vi "Test - Draw Teapot.vi"() -> ()   [LabVIEW 2022 SP3, in "Raster.lvlib"] (continued)
 "Alpha Blending Enabled"=FALSE, "Colour"=131841}, {"Vertex 1"={"Position"={"x"=297.17767, "y"=396.39102, "z"=0.98972005}, "UV"={"u"=0.0, "v"=0.0}, "Colour"=12517256}, "Vertex 2"={"Position"={"x"=313.01276, "y"=398.35367, "z"=0.9897707}, "UV"={"u"=0.0, "v"=0.0}, "Colour"=12517256}, "Vertex 3"={"Position"={"x"=314.0461, "y"=401.00818, "z"=0.9894933}, "UV"={"u"=0.0, "v"=0.0}, "Colour"=12517256}, "Alpha"=0.0, "Alpha Blending Enabled"=FALSE, "Colour"=9091426}, {"Vertex 1"={"Position"={"x"=719.345, "y"=369.09378, "z"=0.9897083}, "UV"={"u"=0.0, "v"=0.0}, "Colour"=12517256}, "Vertex 2"={"Position"={"x"=706.15826, "y"=351.93036, "z"=0.9896661}, "UV"={"u"=0.0, "v"=0.0}, "Colour"=12517256}, "Vertex 3"={"Position"={"x"=702.0343, "y"=353.5881, "z"=0.98960906}, "UV"={"u"=0.0, "v"=0.0}, "Colour"=12517256}, "Alpha"=0.0, "Alpha Blending Enabled"=FALSE, "Colour"=5995329}, {"Vertex 1"={"Position"={"x"=682.03534, "y"=357.63016, "z"=0.9896661}, "UV"={"u"=0.0, "v"=0.0}, "Colour"=12517256}, "Vertex 2"={"Position"={"x"=677.0391, "y"=342.4919, "z"=0.9896034}, "UV"={"u"=0.0, "v"=0.0}, "Colour"=12517256}, "Vertex 3"={"Position"={"x"=669.9876, "y"=344.076, "z"=0.9897131}, "UV"={"u"=0.0, "v"=0.0}, "Colour"=12517256}, "Alpha"=0.0, "Alpha Blending Enabled"=FALSE, "Colour"=9354853}, {"Vertex 1"={"Position"={"x"=402.95343, "y"=420.3544, "z"=0.98970723}, "UV"={"u"=0.0, "v"=0.0}, "Colour"=12517256}, "Vertex 2"={"Position"={"x"=403.55054, "y"=415.85388, "z"=0.98963785}, "UV"={"u"=0.0, "v"=0.0}, "Colour"=12517256}, "Vertex 3"={"Position"={"x"=400.0, "y"=415.91602, "z"=0.9896323}, "UV"={"u"=0.0, "v"=0.0}, "Colour"=12517256}, "Alpha"=0.0, "Alpha Blending Enabled"=FALSE, "Colour"=12253573}, {"Vertex 1"={"Position"={"x"=221.27509, "y"=350.14075, "z"=0.9894772}, "UV"={"u"=0.0, "v"=0.0}, "Colour"=12517256}, "Vertex 2"={"Position"={"x"=213.20128, "y"=333.07422, "z"=0.9894514}, "UV"={"u"=0.0, "v"=0.0}, "Colour"=12517256}, "Vertex 3"={"Position"={"x"=221.4342, "y"=331.2093, "z"=0.990049}, "UV"={"u"=0.0, "v"=0.0}, "Colour"=12517256}, "Alpha"=0.0, "Alpha Blending Enabled"=FALSE, "Colour"=4282158}, {"Vertex 1"={"Position"={"x"=586.7987, "y"=333.07422, "z"=0.9894514}, "UV"={"u"=0.0, "v"=0.0}, "Colour"=12517256}, "Vertex 2"={"Position"={"x"=578.7249, "y"=350.14075, "z"=0.9894772}, "UV"={"u"=0.0, "v"=0.0}, "Colour"=12517256}, "Vertex 3"={"Position"={"x"=571.2652, "y"=347.42908, "z"=0.990049}, "UV"={"u"=0.0, "v"=0.0}, "Colour"=12517256}, "Alpha"=0.0, "Alpha Blending Enabled"=FALSE, "Colour"=4282158}, {"Vertex 1"={"Position"={"x"=373.0144, "y"=460.57834, "z"=0.9896675}, "UV"={"u"=0.0, "v"=0.0}, "Colour"=12517256}, "Vertex 2"={"Position"={"x"=368.50552, "y"=457.60767, "z"=0.98960376}, "UV"={"u"=0.0, "v"=0.0}, "Colour"=12517256}, "Vertex 3"={"Position"={"x"=365.71857, "y"=456.0784, "z"=0.9897051}, "UV"={"u"=0.0, "v"=0.0}, "Colour"=12517256}, "Alpha"=0.0, "Alpha Blending Enabled"=FALSE, "Colour"=9881963}, {"Vertex 1"={"Position"={"x"=706.8331, "y"=370.62793, "z"=0.9896408}, "UV"={"u"=0.0, "v"=0.0}, "Colour"=12517256}, "Vertex 2"={"Position"={"x"=723.916, "y"=383.22333, "z"=0.9896593}, "UV"={"u"=0.0, "v"=0.0}, "Colour"=12517256}, "Vertex 3"={"Position"={"x"=732.98505, "y"=383.09384, "z"=0.9896755}, "UV"={"u"=0.0, "v"=0.0}, "Colour"=12517256}, "Alpha"=0.0, "Alpha Blending Enabled"=FALSE, "Colour"=8432732}, {"Vertex 1"={"Position"={"x"=702.0343, "y"=353.5881, "z"=0.98960906}, "UV"={"u"=0.0, "v"=0.0}, "Colour"=12517256}, "Vertex 2"={"Position"={"x"=713.92786, "y"=369.94937, "z"=0.9896577}, "UV"={"u"=0.0, "v"=0.0}, "Colour"=12517256}, "Vertex 3"={"Position"={"x"=719.345, "y"=369.09378, "z"=0.9897083}, "UV"={"u"=0.0, "v"=0.0}, "Colour"=12517256}, "Alpha"=0.0, "Alpha Blending Enabled"=FALSE, "Colour"=7115086}, {"Vertex 1"={"Position"={"x"=391.0851, "y"=426.15314, "z"=0.9897195}, "UV"={"u"=0.0, "v"=0.0}, "Colour"=12517256}, "Vertex 2"={"Position"={"x"=388.97626, "y"=433.47845, "z"=0.9896417}, "UV"={"u"=0.0, "v"=0.0}, "Colour"=12517256}, "Vertex 3"={"Position"={"x"=392.3791, "y"=433.84442, "z"=0.9896132}, "UV"={"u"=0.0, "v"=0.0}, "Colour"=12517256}, "Alpha"=0.0, "Alpha Blending Enabled"=FALSE, "Colour"=1712915}, {"Vertex 1"={"Position"={"x"=396.07202, "y"=434.0735, "z"=0.9895953}, "UV"={"u"=0.0, "v"=0.0}, "Colour"=12517256}, "Vertex 2"={"Position"={"x"=396.8272, "y"=426.60828, "z"=0.9896822}, "UV"={"u"=0.0, "v"=0.0}, "Colour"=12517256}, "Vertex 3"={"Position"={"x"=393.84116, "y"=426.43307, "z"=0.98969656}, "UV"={"u"=0.0, "v"=0.0}, "Colour"=12517256}, "Alpha"=0.0, "Alpha Blending Enabled"=FALSE, "Colour"=2107927}, {"Vertex 1"={"Position"={"x"=732.98505, "y"=383.09384, "z"=0.9896755}, "UV"={"u"=0.0, "v"=0.0}, "Colour"=12517256}, "Vertex 2"={"Position"={"x"=713.92786, "y"=369.94937, "z"=0.9896577}, "UV"={"u"=0.0, "v"=0.0}, "Colour"=12517256}, "Vertex 3"={"Position"={"x"=706.8331, "y"=370.62793, "z"=0.9896408}, "UV"={"u"=0.0, "v"=0.0}, "Colour"=12517256}, "Alpha"=0.0, "Alpha Blending Enabled"=FALSE, "Colour"=7971671}, {"Vertex 1"={"Position"={"x"=400.0, "y"=420.40808, "z"=0.9897026}, "UV"={"u"=0.0, "v"=0.0}, "Colour"=12517256}, "Vertex 2"={"Position"={"x"=400.0, "y"=415.91602, "z"=0.9896323}, "UV"={"u"=0.0, "v"=0.0}, "Colour"=12517256}, "Vertex 3"={"Position"={"x"=396.44946, "y"=415.85388, "z"=0.98963785}, "UV"={"u"=0.0, "v"=0.0}, "Colour"=12517256}, "Alpha"=0.0, "Alpha Blending Enabled"=FALSE, "Colour"=12253573}, {"Vertex 1"={"Position"={"x"=666.5026, "y"=329.28787, "z"=0.9896555}, "UV"={"u"=0.0, "v"=0.0}, "Colour"=12517256}, "Vertex 2"={"Position"={"x"=669.9876, "y"=344.076, "z"=0.9897131}, "UV"={"u"=0.0, "v"=0.0}, "Colour"=12517256}, "Vertex 3"={"Position"={"x"=677.0391, "y"=342.4919, "z"=0.9896034}, "UV"={"u"=0.0, "v"=0.0}, "Colour"=12517256}, "Alpha"=0.0, "Alpha Blending Enabled"=FALSE, "Colour"=8827744}, {"Vertex 1"={"Position"={"x"=381.9381, "y"=412.10922, "z"=0.98957527}, "UV"={"u"=0.0, "v"=0.0}, "Colour"=12517256}, "Vertex 2"={"Position"={"x"=387.2426, "y"=415.00214, "z"=0.98971444}, "UV"={"u"=0.0, "v"=0.0}, "Colour"=12517256}, "Vertex 3"={"Position"={"x"=390.02243, "y"=415.3864, "z"=0.9896799}, "UV"={"u"=0.0, "v"=0.0}, "Colour"=12517256}, "Alpha"=0.0, "Alpha Blending Enabled"=FALSE, "Colour"=11331451}, {"Vertex 1"={"Position"={"x"=415.18842, "y"=414.5321, "z"=0.9897567}, "UV"={"u"=0.0, "v"=0.0}, "Colour"=12517256}, "Vertex 2"={"Position"={"x"=421.46735, "y"=411.46152, "z"=0.9896358}, "UV"={"u"=0.0, "v"=0.0}, "Colour"=12517256}, "Vertex 3"={"Position"={"x"=418.06192, "y"=412.10922, "z"=0.98957527}, "UV"={"u"=0.0, "v"=0.0}, "Colour"=12517256}, "Alpha"=0.0, "Alpha Blending Enabled"=FALSE, "Colour"=10936183}, {"Vertex 1"={"Position"={"x"=678.03265, "y"=257.92834, "z"=0.98976254}, "UV"={"u"=0.0, "v"=0.0}, "Colour"=12517256}, "Vertex 2"={"Position"={"x"=666.5512, "y"=236.05386, "z"=0.9897306}, "UV"={"u"=0.0, "v"=0.0}, "Colour"=12517256}, "Vertex 3"={"Position"={"x"=671.18396, "y"=239.12437, "z"=0.9894685}, "UV"={"u"=0.0, "v"=0.0}, "Colour"=12517256}, "Alpha"=0.0, "Alpha Blending Enabled"=FALSE, "Colour"=131841}, {"Vertex 1"={"Position"={"x"=723.916, "y"=383.22333, "z"=0.9896593}, "UV"={"u"=0.0, "v"=0.0}, "Colour"=12517256}, "Vertex 2"={"Position"={"x"=706.8331, "y"=370.62793, "z"=0.9896408}, "UV"={"u"=0.0, "v"=0.0}, "Colour"=12517256}, "Vertex 3"={"Position"={"x"=698.73804, "y"=371.07614, "z"=0.9896577}, "UV"={"u"=0.0, "v"=0.0}, "Colour"=12517256}, "Alpha"=0.0, "Alpha Blending Enabled"=FALSE, "Colour"=10409073}, {"Vertex 1"={"Position"={"x"=383.24374, "y"=432.39114, "z"=0.98972654}, "UV"={"u"=0.0, "v"=0.0}, "Colour"=12517256}, "Vertex 2"={"Position"={"x"=378.97202, "y"=439.917, "z"=0.9896443}, "UV"={"u"=0.0, "v"=0.0}, "Colour"=12517256}, "Vertex 3"={"Position"={"x"=382.30276, "y"=440.7109, "z"=0.9895852}, "UV"={"u"=0.0, "v"=0.0}, "Colour"=12517256}, "Alpha"=0.0, "Alpha Blending Enabled"=FALSE, "Colour"=131841}, {"Vertex 1"={"Position"={"x"=209.53932, "y"=162.75063, "z"=0.9894397}, "UV"={"u"=0.0, "v"=0.0}, "Colour"=12517256}, "Vertex 2"={"Position"={"x"=218.06183, "y"=155.67198, "z"=0.9894669}, "UV"={"u"=0.0, "v"=0.0}, "Colour"=12517256}, "Vertex 3"={"Position"={"x"=225.82498, "y"=163.60995, "z"=0.990049}, "UV"={"u"=0.0, "v"=0.0}, "Colour"=12517256}, "Alpha"=0.0, "Alpha Blending Enabled"=FALSE, "Colour"=131841}, {"Vertex 1"={"Position"={"x"=581.9382, "y"=155.67198, "z"=0.9894669}, "UV"={"u"=0.0, "v"=0.0}, "Colour"=12517256}, "Vertex 2"={"Position"={"x"=590.4607, "y"=162.75063, "z"=0.9894397}, "UV"={"u"=0.0, "v"=0.0}, "Colour"=12517256}, "Vertex 3"={"Position"={"x"=581.86536, "y"=170.63258, "z"=0.990049}, "UV"={"u"=0.0, "v"=0.0}, "Colour"=12517256}, "Alpha"=0.0, "Alpha Blending Enabled"=FALSE, "Colour"=131841}, {"Vertex 1"={"Position"={"x"=428.45627, "y"=446.1597, "z"=0.9896467}, "UV"={"u"=0.0, "v"=0.0}, "Colour"=12517256}, "Vertex 2"={"Position"={"x"=431.51227, "y"=452.57986, "z"=0.9896035}, "UV"={"u"=0.0, "v"=0.0}, "Colour"=12517256}, "Vertex 3"={"Position"={"x"=434.30084, "y"=451.0985, "z"=0.98970497}, "UV"={"u"=0.0, "v"=0.0}, "Colour"=12517256}, "Alpha"=0.0, "Alpha Blending Enabled"=FALSE, "Colour"=131841}, {"Vertex 1"={"Position"={"x"=403.92798, "y"=434.0735, "z"=0.9895953}, "UV"={"u"=0.0, "v"=0.0}, "Colour"=12517256}, "Vertex 2"={"Position"={"x"=403.1728, "y"=426.60828, "z"=0.9896822}, "UV"={"u"=0.0, "v"=0.0}, "Colour"=12517256}, "Vertex 3"={"Position"={"x"=400.0, "y"=426.66876, "z"=0.98967725}, "UV"={"u"=0.0, "v"=0.0}, "Colour"=12517256}, "Alpha"=0.0, "Alpha Blending Enabled"=FALSE, "Colour"=2240025}, {"Vertex 1"={"Position"={"x"=406.1588, "y"=426.43307, "z"=0.98969656}, "UV"={"u"=0.0, "v"=0.0}, "Colour"=12517256}, "Vertex 2"={"Position"={"x"=407.6209, "y"=433.84442, "z"=0.9896132}, "UV"={"u"=0.0, "v"=0.0}, "Colour"=12517256}, "Vertex 3"={"Position"={"x"=411.0237, "y"=433.47845, "z"=0.9896417}, "UV"={"u"=0.0, "v"=0.0}, "Colour"=12517256}, "Alpha"=0.0, "Alpha Blending Enabled"=FALSE, "Colour"=1712915}, {"Vertex 1"={"Position"={"x"=400.0, "y"=434.1526, "z"=0.9895892}, "UV"={"u"=0.0, "v"=0.0}, "Colour"=12517256}, "Vertex 2"={"Position"={"x"=400.0, "y"=426.66876, "z"=0.98967725}, "UV"={"u"=0.0, "v"=0.0}, "Colour"=12517256}, "Vertex 3"={"Position"={"x"=396.8272, "y"=426.60828, "z"=0.9896822}, "UV"={"u"=0.0, "v"=0.0}, "Colour"=12517256}, "Alpha"=0.0, "Alpha Blending Enabled"=FALSE, "Colour"=2240025}, {"Vertex 1"={"Position"={"x"=326.15854, "y"=127.58133, "z"=0.9898128}, "UV"={"u"=0.0, "v"=0.0}, "Colour"=12517256}, "Vertex 2"={"Position"={"x"=299.14365, "y"=127.179695, "z"=0.98972636}, "UV"={"u"=0.0, "v"=0.0}, "Colour"=12517256}, "Vertex 3"={"Position"={"x"=299.91116, "y"=121.74838, "z"=0.98940194}, "UV"={"u"=0.0, "v"=0.0}, "Colour"=12517256}, "Alpha"=0.0, "Alpha Blending Enabled"=FALSE, "Colour"=131841}, {"Vertex 1"={"Position"={"x"=375.695, "y"=410.7137, "z"=0.9897057}, "UV"={"u"=0.0, "v"=0.0}, "Colour"=12517256}, "Vertex 2"={"Position"={"x"=365.49564, "y"=408.5937, "z"=0.9895617}, "UV"={"u"=0.0, "v"=0.0}, "Colour"=12517256}, "Vertex 3"={"Position"={"x"=362.46423, "y"=407.4392, "z"=0.98967314}, "UV"={"u"=0.0, "v"=0.0}, "Colour"=12517256}, "Alpha"=0.0, "Alpha Blending Enabled"=FALSE, "Colour"=9816171}, {"Vertex 1"={"Position"={"x"=379.9003, "y"=462.82288, "z"=0.98952234}, "UV"={"u"=0.0, "v"=0.0}, "Colour"=12517256}, "Vertex 2"={"Position"={"x"=387.57538, "y"=462.27194, "z"=0.98972344}, "UV"={"u"=0.0, "v"=0.0}, "Colour"=12517256}, "Vertex 3"={"Position"={"x"=390.27826, "y"=462.79736, "z"=0.98969}, "UV"={"u"=0.0, "v"=0.0}, "Colour"=12517256}, "Alpha"=0.0, "Alpha Blending Enabled"=FALSE, "Colour"=10211439}, {"Vertex 1"={"Position"={"x"=698.73804, "y"=371.07614, "z"=0.9896577}, "UV"={"u"=0.0, "v"=0.0}, "Colour"=12517256}, "Vertex 2"={"Position"={"x"=689.394, "y"=356.5748, "z"=0.98960906}, "UV"={"u"=0.0, "v"=0.0}, "Colour"=12517256}, "Vertex 3"={"Position"={"x"=682.03534, "y"=357.63016, "z"=0.9896661}, "UV"={"u"=0.0, "v"=0.0}, "Colour"=12517256}, "Alpha"=0.0, "Alpha Blending Enabled"=FALSE, "Colour"=11001976}, {"Vertex 1"={"Position"={"x"=213.20128, "y"=333.07422, "z"=0.9894514}, "UV"={"u"=0.0, "v"=0.0}, "Colour"=12517256}, "Vertex 2"={"Position"={"x"=205.60883, "y"=316.07062, "z"=0.9894271}, "UV"={"u"=0.0, "v"=0.0}, "Colour"=12517256}, "Vertex 3"={"Position"={"x"=214.60127, "y"=315.1298, "z"=0.990049}, "UV"={"u"=0.0, "v"=0.0}, "Colour"=12517256}, "Alpha"=0.0, "Alpha Blending Enabled"=FALSE, "Colour"=4084524}, {"Vertex 1"={"Position"={"x"=594.3912, "y"=316.07062, "z"=0.9894271}, "UV"={"u"=0.0, "v"=0.0}, "Colour"=12517256}, "Vertex 2"={"Position"={"x"=586.7987, "y"=333.07422, "z"=0.9894514}, "UV"={"u"=0.0, "v"=0.0}, "Colour"=12517256}, "Vertex 3"={"Position"={"x"=578.5658, "y"=331.2093, "z"=0.990049}, "UV"={"u"=0.0, "v"=0.0}, "Colour"=12517256}, "Alpha"=0.0, "Alpha Blending Enabled"=FALSE, "Colour"=4084524}, {"Vertex 1"={"Position"={"x"=387.2426, "y"=415.00214, "z"=0.98971444}, "UV"={"u"=0.0, "v"=0.0}, "Colour"=12517256}, "Vertex 2"={"Position"={"x"=381.9381, "y"=412.10922, "z"=0.98957527}, "UV"={"u"=0.0, "v"=0.0}, "Colour"=12517256}, "Vertex 3"={"Position"={"x"=378.53265, "y"=411.46152, "z"=0.9896358}, "UV"={"u"=0.0, "v"=0.0}, "Colour"=12517256}, "Alpha"=0.0, "Alpha Blending Enabled"=FALSE, "Colour"=10936183}, {"Vertex 1"={"Position"={"x"=376.19745, "y"=438.9993, "z"=0.9897126}, "UV"={"u"=0.0, "v"=0.0}, "Colour"=12517256}, "Vertex 2"={"Position"={"x"=371.54373, "y"=446.1597, "z"=0.9896467}, "UV"={"u"=0.0, "v"=0.0}, "Colour"=12517256}, "Vertex 3"={"Position"={"x"=374.82742, "y"=447.3146, "z"=0.98956454}, "UV"={"u"=0.0, "v"=0.0}, "Colour"=12517256}, "Alpha"=0.0, "Alpha Blending Enabled"=FALSE, "Colour"=131841}, {"Vertex 1"={"Position"={"x"=374.82742, "y"=447.3146, "z"=0.98956454}, "UV"={"u"=0.0, "v"=0.0}, "Colour"=12517256}, "Vertex 2"={"Position"={"x"=378.97202, "y"=439.917, "z"=0.9896443}, "UV"={"u"=0.0, "v"=0.0}, "Colour"=12517256}, "Vertex 3"={"Position"={"x"=376.19745, "y"=438.9993, "z"=0.9897126}, "UV"={"u"=0.0, "v"=0.0}, "Colour"=12517256}, "Alpha"=0.0, "Alpha Blending Enabled"=FALSE, "Colour"=131841}, {"Vertex 1"={"Position"={"x"=414.14594, "y"=412.64026, "z"=0.98952574}, "UV"={"u"=0.0, "v"=0.0}, "Colour"=12517256}, "Vertex 2"={"Position"={"x"=409.97757, "y"=415.3864, "z"=0.9896799}, "UV"={"u"=0.0, "v"=0.0}, "Colour"=12517256}, "Vertex 3"={"Position"={"x"=412.75735, "y"=415.00214, "z"=0.98971444}, "UV"={"u"=0.0, "v"=0.0}, "Colour"=12517256}, "Alpha"=0.0, "Alpha Blending Enabled"=FALSE, "Colour"=11331451}, {"Vertex 1"={"Position"={"x"=682.01483, "y"=260.7837, "z"=0.9895282}, "UV"={"u"=0.0, "v"=0.0}, "Colour"=12517256}, "Vertex 2"={"Position"={"x"=688.6595, "y"=283.87192, "z"=0.9895922}, "UV"={"u"=0.0, "v"=0.0}, "Colour"=12517256}, "Vertex 3"={"Position"={"x"=685.4334, "y"=281.3033, "z"=0.9897971}, "UV"={"u"=0.0, "v"=0.0}, "Colour"=12517256}, "Alpha"=0.0, "Alpha Blending Enabled"=FALSE, "Colour"=131841}, {"Vertex 1"={"Position"={"x"=485.95386, "y"=401.00818, "z"=0.9894933}, "UV"={"u"=0.0, "v"=0.0}, "Colour"=12517256}, "Vertex 2"={"Position"={"x"=469.47156, "y"=402.4644, "z"=0.9895999}, "UV"={"u"=0.0, "v"=0.0}, "Colour"=12517256}, "Vertex 3"={"Position"={"x"=470.66293, "y"=400.277, "z"=0.989823}, "UV"={"u"=0.0, "v"=0.0}, "Colour"=12517256}, "Alpha"=0.0, "Alpha Blending Enabled"=FALSE, "Colour"=9091426}, {"Vertex 1"={"Position"={"x"=431.51227, "y"=452.57986, "z"=0.9896035}, "UV"={"u"=0.0, "v"=0.0}, "Colour"=12517256}, "Vertex 2"={"Position"={"x"=431.49448, "y"=457.60767, "z"=0.98960376}, "UV"={"u"=0.0, "v"=0.0}, "Colour"=12517256}, "Vertex 3"={"Position"={"x"=434.28143, "y"=456.0784, "z"=0.9897051}, "UV"={"u"=0.0, "v"=0.0}, "Colour"=12517256}, "Alpha"=0.0, "Alpha Blending Enabled"=FALSE, "Colour"=4677427}, {"Vertex 1"={"Position"={"x"=362.46423, "y"=407.4392, "z"=0.98967314}, "UV"={"u"=0.0, "v"=0.0}, "Colour"=12517256}, "Vertex 2"={"Position"={"x"=348.88834, "y"=405.76608, "z"=0.98953724}, "UV"={"u"=0.0, "v"=0.0}, "Colour"=12517256}, "Vertex 3"={"Position"={"x"=346.3009, "y"=404.1098, "z"=0.98970187}, "UV"={"u"=0.0, "v"=0.0}, "Colour"=12517256}, "Alpha"=0.0, "Alpha Blending Enabled"=FALSE, "Colour"=9355110}, {"Vertex 1"={"Position"={"x"=368.50552, "y"=457.60767, "z"=0.98960376}, "UV"={"u"=0.0, "v"=0.0}, "Colour"=12517256}, "Vertex 2"={"Position"={"x"=368.48776, "y"=452.57986, "z"=0.9896035}, "UV"={"u"=0.0, "v"=0.0}, "Colour"=12517256}, "Vertex 3"={"Position"={"x"=365.69916, "y"=451.0985, "z"=0.98970497}, "UV"={"u"=0.0, "v"=0.0}, "Colour"=12517256}, "Alpha"=0.0, "Alpha Blending Enabled"=FALSE, "Colour"=4677427}, {"Vertex 1"={"Position"={"x"=192.4563, "y"=195.83786, "z"=0.9896561}, "UV"={"u"=0.0, "v"=0.0}, "Colour"=12517256}, "Vertex 2"={"Position"={"x"=171.12422, "y"=206.32034, "z"=0.9896561}, "UV"={"u"=0.0, "v"=0.0}, "Colour"=12517256}, "Vertex 3"={"Position"={"x"=169.41815, "y"=209.785, "z"=0.98959744}, "UV"={"u"=0.0, "v"=0.0}, "Colour"=12517256}, "Alpha"=0.0, "Alpha Blending Enabled"=FALSE, "Colour"=1515280}, {"Vertex 1"={"Position"={"x"=169.40346, "y"=222.90483, "z"=0.9896561}, "UV"={"u"=0.0, "v"=0.0}, "Colour"=12517256}, "Vertex 2"={"Position"={"x"=186.3216, "y"=214.24203, "z"=0.9896561}, "UV"={"u"=0.0, "v"=0.0}, "Colour"=12517256}, "Vertex 3"={"Position"={"x"=186.59279, "y"=209.32652, "z"=0.98959744}, "UV"={"u"=0.0, "v"=0.0}, "Colour"=12517256}, "Alpha"=0.0, "Alpha Blending Enabled"=FALSE, "Colour"=11858305}, {"Vertex 1"={"Position"={"x"=171.12422, "y"=206.32034, "z"=0.9896561}, "UV"={"u"=0.0, "v"=0.0}, "Colour"=12517256}, "Vertex 2"={"Position"={"x"=152.20497, "y"=217.41687, "z"=0.9896561}, "UV"={"u"=0.0, "v"=0.0}, "Colour"=12517256}, "Vertex 3"={"Position"={"x"=151.36185, "y"=220.60233, "z"=0.98959744}, "UV"={"u"=0.0, "v"=0.0}, "Colour"=12517256}, "Alpha"=0.0, "Alpha Blending Enabled"=FALSE, "Colour"=1778707}, {"Vertex 1"={"Position"={"x"=154.51155, "y"=232.58194, "z"=0.9896561}, "UV"={"u"=0.0, "v"=0.0}, "Colour"=12517256}, "Vertex 2"={"Position"={"x"=169.40346, "y"=222.90483, "z"=0.9896561}, "UV"={"u"=0.0, "v"=0.0}, "Colour"=12517256}, "Vertex 3"={"Position"={"x"=168.51642, "y"=218.47636, "z"=0.98959744}, "UV"={"u"=0.0, "v"=0.0}, "Colour"=12517256}, "Alpha"=0.0, "Alpha Blending Enabled"=FALSE, "Colour"=11529085}, {"Vertex 1"={"Position"={"x"=152.20497, "y"=217.41687, "z"=0.9896561}, "UV"={"u"=0.0, "v"=0.0}, "Colour"=12517256}, "Vertex 2"={"Position"={"x"=135.65894, "y"=229.04527, "z"=0.9896561}, "UV"={"u"=0.0, "v"=0.0}, "Colour"=12517256}, "Vertex 3"={"Position"={"x"=135.59482, "y"=232.01439, "z"=0.98959744}, "UV"={"u"=0.0, "v"=0.0}, "Colour"=12517256}, "Alpha"=0.0, "Alpha Blending Enabled"=FALSE, "Colour"=2240024}, {"Vertex 1"={"Position"={"x"=141.58824, "y"=243.03935, "z"=0.9896561}, "UV"={"u"=0.0, "v"=0.0}, "Colour"=12517256}, "Vertex 2"={"Position"={"x"=154.51155, "y"=232.58194, "z"=0.9896561}, "UV"={"u"=0.0, "v"=0.0}, "Colour"=12517256}, "Vertex 3"={"Position"={"x"=152.57072, "y"=228.54994, "z"=0.98959744}, "UV"={"u"=0.0, "v"=0.0}, "Colour"=12517256}, "Alpha"=0.0, "Alpha Blending Enabled"=FALSE, "Colour"=11199609}, {"Vertex 1"={"Position"={"x"=135.65894, "y"=229.04527, "z"=0.9896561}, "UV"={"u"=0.0, "v"=0.0}, "Colour"=12517256}, "Vertex 2"={"Position"={"x"=121.447014, "y"=241.12357, "z"=0.9896561}, "UV"={"u"=0.0, "v"=0.0}, "Colour"=12517256}, "Vertex 3"={"Position"={"x"=122.07298, "y"=243.90215, "z"=0.98959744}, "UV"={"u"=0.0, "v"=0.0}, "Colour"=12517256}, "Alpha"=0.0, "Alpha Blending Enabled"=FALSE, "Colour"=2898719}, {"Vertex 1"={"Position"={"x"=130.57544, "y"=254.04317, "z"=0.9896561}, "UV"={"u"=0.0, "v"=0.0}, "Colour"=12517256}, "Vertex 2"={"Position"={"x"=141.58824, "y"=243.03935, "z"=0.9896561}, "UV"={"u"=0.0, "v"=0.0}, "Colour"=12517256}, "Vertex 3"={"Position"={"x"=138.70209, "y"=239.3482, "z"=0.98959744}, "UV"={"u"=0.0, "v"=0.0}, "Colour"=12517256}, "Alpha"=0.0, "Alpha Blending Enabled"=FALSE, "Colour"=10804341}, {"Vertex 1"={"Position"={"x"=121.447014, "y"=241.12357, "z"=0.9896561}, "UV"={"u"=0.0, "v"=0.0}, "Colour"=12517256}, "Vertex 2"={"Position"={"x"=109.52954, "y"=253.56958, "z"=0.9896561}, "UV"={"u"=0.0, "v"=0.0}, "Colour"=12517256}, "Vertex 3"={"Position"={"x"=110.75225, "y"=256.14658, "z"=0.98959744}, "UV"={"u"=0.0, "v"=0.0}, "Colour"=12517256}, "Alpha"=0.0, "Alpha Blending Enabled"=FALSE, "Colour"=3557415}, {"Vertex 1"={"Position"={"x"=121.415565, "y"=265.35983, "z"=0.9896561}, "UV"={"u"=0.0, "v"=0.0}, "Colour"=12517256}, "Vertex 2"={"Position"={"x"=130.57544, "y"=254.04317, "z"=0.9896561}, "UV"={"u"=0.0, "v"=0.0}, "Colour"=12517256}, "Vertex 3"={"Position"={"x"=126.85683, "y"=250.67299, "z"=0.98959744}, "UV"={"u"=0.0, "v"=0.0}, "Colour"=12517256}, "Alpha"=0.0, "Alpha Blending Enabled"=FALSE, "Colour"=10409073}, {"Vertex 1"={"Position"={"x"=109.52954, "y"=253.56958, "z"=0.9896561}, "UV"={"u"=0.0, "v"=0.0}, "Colour"=12517256}, "Vertex 2"={"Position"={"x"=99.86725, "y"=266.30142, "z"=0.9896561}, "UV"={"u"=0.0, "v"=0.0}, "Colour"=12517256}, "Vertex 3"={"Position"={"x"=101.588585, "y"=268.6284, "z"=0.98959744}, "UV"={"u"=0.0, "v"=0.0}, "Colour"=12517256}, "Alpha"=0.0, "Alpha Blending Enabled"=FALSE, "Colour"=4216366}, {"Vertex 1"={"Position"={"x"=114.0508, "y"=276.7551, "z"=0.9896561}, "UV"={"u"=0.0, "v"=0.0}, "Colour"=12517256}, "Vertex 2"={"Position"={"x"=121.415565, "y"=265.35983, "z"=0.9896561}, "UV"={"u"=0.0, "v"=0.0}, "Colour"=12517256}, "Vertex 3"={"Position"={"x"=116.981316, "y"=262.32532, "z"=0.98959744}, "UV"={"u"=0.0, "v"=0.0}, "Colour"=12517256}, "Alpha"=0.0, "Alpha Blending Enabled"=FALSE, "Colour"=9948012}, {"Vertex 1"={"Position"={"x"=99.86725, "y"=266.30142, "z"=0.9896561}, "UV"={"u"=0.0, "v"=0.0}, "Colour"=12517256}, "Vertex 2"={"Position"={"x"=92.42079, "y"=279.23703, "z"=0.9896561}, "UV"={"u"=0.0, "v"=0.0}, "Colour"=12517256}, "Vertex 3"={"Position"={"x"=94.53805, "y"=281.22873, "z"=0.98959744}, "UV"={"u"=0.0, "v"=0.0}, "Colour"=12517256}, "Alpha"=0.0, "Alpha Blending Enabled"=FALSE, "Colour"=4940853}, {"Vertex 1"={"Position"={"x"=108.42314, "y"=287.9951, "z"=0.9896561}, "UV"={"u"=0.0, "v"=0.0}, "Colour"=12517256}, "Vertex 2"={"Position"={"x"=114.0508, "y"=276.7551, "z"=0.9896561}, "UV"={"u"=0.0, "v"=0.0}, "Colour"=12517256}, "Vertex 3"={"Position"={"x"=109.02176, "y"=274.10672, "z"=0.98959744}, "UV"={"u"=0.0, "v"=0.0}, "Colour"=12517256}, "Alpha"=0.0, "Alpha Blending Enabled"=FALSE, "Colour"=9552487}, {"Vertex 1"={"Position"={"x"=92.42079, "y"=279.23703, "z"=0.9896561}, "UV"={"u"=0.0, "v"=0.0}, "Colour"=12517256}, "Vertex 2"={"Position"={"x"=87.15057, "y"=292.2944, "z"=0.9896561}, "UV"={"u"=0.0, "v"=0.0}, "Colour"=12517256}, "Vertex 3"={"Position"={"x"=89.5565, "y"=293.82855, "z"=0.98959744}, "UV"={"u"=0.0, "v"=0.0}, "Colour"=12517256}, "Alpha"=0.0, "Alpha Blending Enabled"=FALSE, "Colour"=5599805}, {"Vertex 1"={"Position"={"x"=104.47511, "y"=298.84622, "z"=0.9896561}, "UV"={"u"=0.0, "v"=0.0}, "Colour"=12517256}, "Vertex 2"={"Position"={"x"=108.42314, "y"=287.9951, "z"=0.9896561}, "UV"={"u"=0.0, "v"=0.0}, "Colour"=12517256}, "Vertex 3"={"Position"={"x"=102.92444, "y"=285.8186, "z"=0.98959744}, "UV"={"u"=0.0, "v"=0.0}, "Colour"=12517256}, "Alpha"=0.0, "Alpha Blending Enabled"=FALSE, "Colour"=9025634}, {"Vertex 1"={"Position"={"x"=87.15057, "y"=292.2944, "z"=0.9896561}, "UV"={"u"=0.0, "v"=0.0}, "Colour"=12517256}, "Vertex 2"={"Position"={"x"=84.01742, "y"=305.39136, "z"=0.9896561}, "UV"={"u"=0.0, "v"=0.0}, "Colour"=12517256}, "Vertex 3"={"Position"={"x"=86.5999, "y"=306.30865, "z"=0.98959744}, "UV"={"u"=0.0, "v"=0.0}, "Colour"=12517256}, "Alpha"=0.0, "Alpha Blending Enabled"=FALSE, "Colour"=6258756}, {"Vertex 1"={"Position"={"x"=102.14853, "y"=309.0745, "z"=0.9896561}, "UV"={"u"=0.0, "v"=0.0}, "Colour"=12517256}, "Vertex 2"={"Position"={"x"=104.47511, "y"=298.84622, "z"=0.9896561}, "UV"={"u"=0.0, "v"=0.0}, "Colour"=12517256}, "Vertex 3"={"Position"={"x"=98.63565, "y"=297.2621, "z"=0.98959744}, "UV"={"u"=0.0, "v"=0.0}, "Colour"=12517256}, "Alpha"=0.0, "Alpha Blending Enabled"=FALSE, "Colour"=8432732}, {"Vertex 1"={"Position"={"x"=84.01742, "y"=305.39136, "z"=0.9896561}, "UV"={"u"=0.0, "v"=0.0}, "Colour"=12517256}, "Vertex 2"={"Position"={"x"=82.98175, "y"=318.44592, "z"=0.9896561}, "UV"={"u"=0.0, "v"=0.0}, "Colour"=12517256}, "Vertex 3"={"Position"={"x"=85.62412, "y"=318.55002, "z"=0.98959744}, "UV"={"u"=0.0, "v"=0.0}, "Colour"=12517256}, "Alpha"=0.0, "Alpha Blending Enabled"=FALSE, "Colour"=6983244}, {"Vertex 1"={"Position"={"x"=101.3859, "y"=318.44592, "z"=0.9896561}, "UV"={"u"=0.0, "v"=0.0}, "Colour"=12517256}, "Vertex 2"={"Position"={"x"=102.14853, "y"=309.0745, "z"=0.9896561}, "UV"={"u"=0.0, "v"=0.0}, "Colour"=12517256}, "Vertex 3"={"Position"={"x"=96.10178, "y"=308.23883, "z"=0.98959744}, "UV"={"u"=0.0, "v"=0.0}, "Colour"=12517256}, "Alpha"=0.0, "Alpha Blending Enabled"=FALSE, "Colour"=7773780}, {"Vertex 1"={"Position"={"x"=82.98175, "y"=318.44592, "z"=0.9896561}, "UV"={"u"=0.0, "v"=0.0}, "Colour"=12517256}, "Vertex 2"={"Position"={"x"=84.52947, "y"=330.19464, "z"=0.9896561}, "UV"={"u"=0.0, "v"=0.0}, "Colour"=12517256}, "Vertex 3"={"Position"={"x"=87.13484, "y"=329.46445, "z"=0.98959744}, "UV"={"u"=0.0, "v"=0.0}, "Colour"=12517256}, "Alpha"=0.0, "Alpha Blending Enabled"=FALSE, "Colour"=8037463}, {"Vertex 1"={"Position"={"x"=102.74355, "y"=326.45404, "z"=0.9896561}, "UV"={"u"=0.0, "v"=0.0}, "Colour"=12517256}, "Vertex 2"={"Position"={"x"=101.3859, "y"=318.44592, "z"=0.9896561}, "UV"={"u"=0.0, "v"=0.0}, "Colour"=12517256}, "Vertex 3"={"Position"={"x"=95.26916, "y"=318.55002, "z"=0.98959744}, "UV"={"u"=0.0, "v"=0.0}, "Colour"=12517256}, "Alpha"=0.0, "Alpha Blending Enabled"=FALSE, "Colour"=6522183}, {"Vertex 1"={"Position"={"x"=84.52947, "y"=330.19464, "z"=0.9896561}, "UV"={"u"=0.0, "v"=0.0}, "Colour"=12517256}, "Vertex 2"={"Position"={"x"=89.163445, "y"=339.60242, "z"=0.9896561}, "UV"={"u"=0.0, "v"=0.0}, "Colour"=12517256}, "Vertex 3"={"Position"={"x"=91.65158, "y"=338.20395, "z"=0.98959744}, "UV"={"u"=0.0, "v"=0.0}, "Colour"=12517256}, "Alpha"=0.0, "Alpha Blending Enabled"=FALSE, "Colour"=9552744}, {"Vertex 1"={"Position"={"x"=106.78244, "y"=332.86646, "z"=0.9896561}, "UV"={"u"=0.0, "v"=0.0}, "Colour"=12517256}, "Vertex 2"={"Position"={"x"=102.74355, "y"=326.45404, "z"=0.9896561}, "UV"={"u"=0.0, "v"=0.0}, "Colour"=12517256}, "Vertex 3"={"Position"={"x"=96.68016, "y"=327.50403, "z"=0.98959744}, "UV"={"u"=0.0, "v"=0.0}, "Colour"=12517256}, "Alpha"=0.0, "Alpha Blending Enabled"=FALSE, "Colour"=4545841}, {"Vertex 1"={"Position"={"x"=89.163445, "y"=339.60242, "z"=0.9896561}, "UV"={"u"=0.0, "v"=0.0}, "Colour"=12517256}, "Vertex 2"={"Position"={"x"=96.86964, "y"=346.92914, "z"=0.9896561}, "UV"={"u"=0.0, "v"=0.0}, "Colour"=12517256}, "Vertex 3"={"Position"={"x"=99.15168, "y"=345.0104, "z"=0.98959744}, "UV"={"u"=0.0, "v"=0.0}, "Colour"=12517256}, "Alpha"=0.0, "Alpha Blending Enabled"=FALSE, "Colour"=10936183}, {"Vertex 1"={"Position"={"x"=113.45179, "y"=337.86047, "z"=0.9896561}, "UV"={"u"=0.0, "v"=0.0}, "Colour"=12517256}, "Vertex 2"={"Position"={"x"=106.78244, "y"=332.86646, "z"=0.9896561}, "UV"={"u"=0.0, "v"=0.0}, "Colour"=12517256}, "Vertex 3"={"Position"={"x"=100.88518, "y"=334.67392, "z"=0.98959744}, "UV"={"u"=0.0, "v"=0.0}, "Colour"=12517256}, "Alpha"=0.0, "Alpha Blending Enabled"=FALSE, "Colour"=2766878}, {"Vertex 1"={"Position"={"x"=96.86964, "y"=346.92914, "z"=0.9896561}, "UV"={"u"=0.0, "v"=0.0}, "Colour"=12517256}, "Vertex 2"={"Position"={"x"=107.63404, "y"=352.43503, "z"=0.9896561}, "UV"={"u"=0.0, "v"=0.0}, "Colour"=12517256}, "Vertex 3"={"Position"={"x"=109.61189, "y"=350.12524, "z"=0.98959744}, "UV"={"u"=0.0, "v"=0.0}, "Colour"=12517256}, "Alpha"=0.0, "Alpha Blending Enabled"=FALSE, "Colour"=11792512}, {"Vertex 1"={"Position"={"x"=122.700836, "y"=341.61334, "z"=0.9896561}, "UV"={"u"=0.0, "v"=0.0}, "Colour"=12517256}, "Vertex 2"={"Position"={"x"=113.45179, "y"=337.86047, "z"=0.9896561}, "UV"={"u"=0.0, "v"=0.0}, "Colour"=12517256}, "Vertex 3"={"Position"={"x"=107.84178, "y"=340.25775, "z"=0.98959744}, "UV"={"u"=0.0, "v"=0.0}, "Colour"=12517256}, "Alpha"=0.0, "Alpha Blending Enabled"=FALSE, "Colour"=1581073}, {"Vertex 1"={"Position"={"x"=107.63404, "y"=352.43503, "z"=0.9896561}, "UV"={"u"=0.0, "v"=0.0}, "Colour"=12517256}, "Vertex 2"={"Position"={"x"=121.44258, "y"=356.38025, "z"=0.9896561}, "UV"={"u"=0.0, "v"=0.0}, "Colour"=12517256}, "Vertex 3"={"Position"={"x"=123.00947, "y"=353.7902, "z"=0.98959744}, "UV"={"u"=0.0, "v"=0.0}, "Colour"=12517256}, "Alpha"=0.0, "Alpha Blending Enabled"=FALSE, "Colour"=12253573}, {"Vertex 1"={"Position"={"x"=134.47885, "y"=344.30252, "z"=0.9896561}, "UV"={"u"=0.0, "v"=0.0}, "Colour"=12517256}, "Vertex 2"={"Position"={"x"=122.700836, "y"=341.61334, "z"=0.9896561}, "UV"={"u"=0.0, "v"=0.0}, "Colour"=12517256}, "Vertex 3"={"Position"={"x"=117.50798, "y"=344.45398, "z"=0.98959744}, "UV"={"u"=0.0, "v"=0.0}, "Colour"=12517256}, "Alpha"=0.0, "Alpha Blending Enabled"=FALSE, "Colour"=988171}, {"Vertex 1"={"Position"={"x"=121.44258, "y"=356.38025, "z"=0.9896561}, "UV"={"u"=0.0, "v"=0.0}, "Colour"=12517256}, "Vertex 2"={"Position"={"x"=138.28133, "y"=359.0247, "z"=0.9896561}, "UV"={"u"=0.0, "v"=0.0}, "Colour"=12517256}, "Vertex 3"={"Position"={"x"=139.3214, "y"=356.247, "z"=0.98959744}, "UV"={"u"=0.0, "v"=0.0}, "Colour"=12517256}, "Alpha"=0.0, "Alpha Blending Enabled"=FALSE, "Colour"=12385671}, {"Vertex 1"={"Position"={"x"=148.73495, "y"=346.1051, "z"=0.9896561}, "UV"={"u"=0.0, "v"=0.0}, "Colour"=12517256}, "Vertex 2"={"Position"={"x"=134.47885, "y"=344.30252, "z"=0.9896561}, "UV"={"u"=0.0, "v"=0.0}, "Colour"=12517256}, "Vertex 3"={"Position"={"x"=129.84137, "y"=347.46066, "z"=0.98959744}, "UV"={"u"=0.0, "v"=0.0}, "Colour"=12517256}, "Alpha"=0.0, "Alpha Blending Enabled"=FALSE, "Colour"=724744}, {"Vertex 1"={"Position"={"x"=138.28133, "y"=359.0247, "z"=0.9896561}, "UV"={"u"=0.0, "v"=0.0}, "Colour"=12517256}, "Vertex 2"={"Position"={"x"=158.13632, "y"=360.62878, "z"=0.9896561}, "UV"={"u"=0.0, "v"=0.0}, "Colour"=12517256}, "Vertex 3"={"Position"={"x"=158.52467, "y"=357.73706, "z"=0.98959744}, "UV"={"u"=0.0, "v"=0.0}, "Colour"=12517256}, "Alpha"=0.0, "Alpha Blending Enabled"=FALSE, "Colour"=12451463}, {"Vertex 1"={"Position"={"x"=165.41827, "y"=347.1984, "z"=0.9896561}, "UV"={"u"=0.0, "v"=0.0}, "Colour"=12517256}, "Vertex 2"={"Position"={"x"=148.73495, "y"=346.1051, "z"=0.9896561}, "UV"={"u"=0.0, "v"=0.0}, "Colour"=12517256}, "Vertex 3"={"Position"={"x"=144.79973, "y"=349.47617, "z"=0.98959744}, "UV"={"u"=0.0, "v"=0.0}, "Colour"=12517256}, "Alpha"=0.0, "Alpha Blending Enabled"=FALSE, "Colour"=658952}, {"Vertex 1"={"Position"={"x"=158.13632, "y"=360.62878, "z"=0.9896561}, "UV"={"u"=0.0, "v"=0.0}, "Colour"=12517256}, "Vertex 2"={"Position"={"x"=180.99356, "y"=361.45255, "z"=0.9896561}, "UV"={"u"=0.0, "v"=0.0}, "Colour"=12517256}, "Vertex 3"={"Position"={"x"=180.59659, "y"=358.50238, "z"=0.98959744}, "UV"={"u"=0.0, "v"=0.0}, "Colour"=12517256}, "Alpha"=0.0, "Alpha Blending Enabled"=FALSE, "Colour"=12517000}, {"Vertex 1"={"Position"={"x"=184.47804, "y"=347.7598, "z"=0.9896561}, "UV"={"u"=0.0, "v"=0.0}, "Colour"=12517256}, "Vertex 2"={"Position"={"x"=165.41827, "y"=347.1984, "z"=0.9896561}, "UV"={"u"=0.0, "v"=0.0}, "Colour"=12517256}, "Vertex 3"={"Position"={"x"=162.341, "y"=350.69873, "z"=0.98959744}, "UV"={"u"=0.0, "v"=0.0}, "Colour"=12517256}, "Alpha"=0.0, "Alpha Blending Enabled"=FALSE, "Colour"=724488}, {"Vertex 1"={"Position"={"x"=180.99356, "y"=361.45255, "z"=0.9896561}, "UV"={"u"=0.0, "v"=0.0}, "Colour"=12517256}, "Vertex 2"={"Position"={"x"=206.83899, "y"=361.75607, "z"=0.9896561}, "UV"={"u"=0.0, "v"=0.0}, "Colour"=12517256}, "Vertex 3"={"Position"={"x"=205.5139, "y"=358.7842, "z"=0.98959744}, "UV"={"u"=0.0, "v"=0.0}, "Colour"=12517256}, "Alpha"=0.0, "Alpha Blending Enabled"=FALSE, "Colour"=12517256}, {"Vertex 1"={"Position"={"x"=205.86348, "y"=347.9667, "z"=0.9896561}, "UV"={"u"=0.0, "v"=0.0}, "Colour"=12517256}, "Vertex 2"={"Position"={"x"=184.47804, "y"=347.7598, "z"=0.9896561}, "UV"={"u"=0.0, "v"=0.0}, "Colour"=12517256}, "Vertex 3"={"Position"={"x"=182.42264, "y"=351.32635, "z"=0.98959744}, "UV"={"u"=0.0, "v"=0.0}, "Colour"=12517256}, "Alpha"=0.0, "Alpha Blending Enabled"=FALSE, "Colour"=724744}, {"Vertex 1"={"Position"={"x"=206.83899, "y"=361.75607, "z"=0.9896561}, "UV"={"u"=0.0, "v"=0.0}, "Colour"=12517256}, "Vertex 2"={"Position"={"x"=235.65857, "y"=361.79938, "z"=0.9896561}, "UV"={"u"=0.0, "v"=0.0}, "Colour"=12517256}, "Vertex 3"={"Position"={"x"=233.2539, "y"=358.82452, "z"=0.98959744}, "UV"={"u"=0.0, "v"=0.0}, "Colour"=12517256}, "Alpha"=0.0, "Alpha Blending Enabled"=FALSE, "Colour"=12517256}, {"Vertex 1"={"Position"={"x"=229.52385, "y"=347.99628, "z"=0.9896561}, "UV"={"u"=0.0, "v"=0.0}, "Colour"=12517256}, "Vertex 2"={"Position"={"x"=205.86348, "y"=347.9667, "z"=0.9896561}, "UV"={"u"=0.0, "v"=0.0}, "Colour"=12517256}, "Vertex 3"={"Position"={"x"=205.00276, "y"=351.5577, "z"=0.98959744}, "UV"={"u"=0.0, "v"=0.0}, "Colour"=12517256}, "Alpha"=0.0, "Alpha Blending Enabled"=FALSE, "Colour"=790536}, {"Vertex 1"={"Position"={"x"=414.08487, "y"=432.98935, "z"=0.9896798}, "UV"={"u"=0.0, "v"=0.0}, "Colour"=12517256}, "Vertex 2"={"Position"={"x"=417.69724, "y"=440.7109, "z"=0.9895852}, "UV"={"u"=0.0, "v"=0.0}, "Colour"=12517256}, "Vertex 3"={"Position"={"x"=421.02798, "y"=439.917, "z"=0.9896443}, "UV"={"u"=0.0, "v"=0.0}, "Colour"=12517256}, "Alpha"=0.0, "Alpha Blending Enabled"=FALSE, "Colour"=131841}, {"Vertex 1"={"Position"={"x"=689.394, "y"=356.5748, "z"=0.98960906}, "UV"={"u"=0.0, "v"=0.0}, "Colour"=12517256}, "Vertex 2"={"Position"={"x"=698.73804, "y"=371.07614, "z"=0.9896577}, "UV"={"u"=0.0, "v"=0.0}, "Colour"=12517256}, "Vertex 3"={"Position"={"x"=706.8331, "y"=370.62793, "z"=0.9896408}, "UV"={"u"=0.0, "v"=0.0}, "Colour"=12517256}, "Alpha"=0.0, "Alpha Blending Enabled"=FALSE, "Colour"=10606707}, {"Vertex 1"={"Position"={"x"=417.69724, "y"=440.7109, "z"=0.9895852}, "UV"={"u"=0.0, "v"=0.0}, "Colour"=12517256}, "Vertex 2"={"Position"={"x"=414.08487, "y"=432.98935, "z"=0.9896798}, "UV"={"u"=0.0, "v"=0.0}, "Colour"=12517256}, 
